vi "Excel - Read Array.vi"(6 "Cluster":T1={"start (-1, -1)"={"row"=-1, "column"=-1}, "end (-1, -1)"={"row"=-1, "column"=-1}}, 7 "name (\"\")":string, 8 "Path":path, 9 "worksheet index (0)":i32) -> (0 "False":bool, 2 "Element 1":string[][](array[string]))   [LabVIEW 2015]
uses:
  <vilib>/addons/_office/excel.llb/Excel Get Data ([str]).vi
  <vilib>/Utility/NIReport.llb/NI_report.lvclass
  <vilib>/Utility/NIReport.llb/Excel/NI_Excel.lvclass
  <vilib>/addons/_office/NI_ReportGenerationToolkit.lvlib
panel:
  in  "error in (no error)":errorcluster
  # "Select a Exel file to be Read and then Press Open"
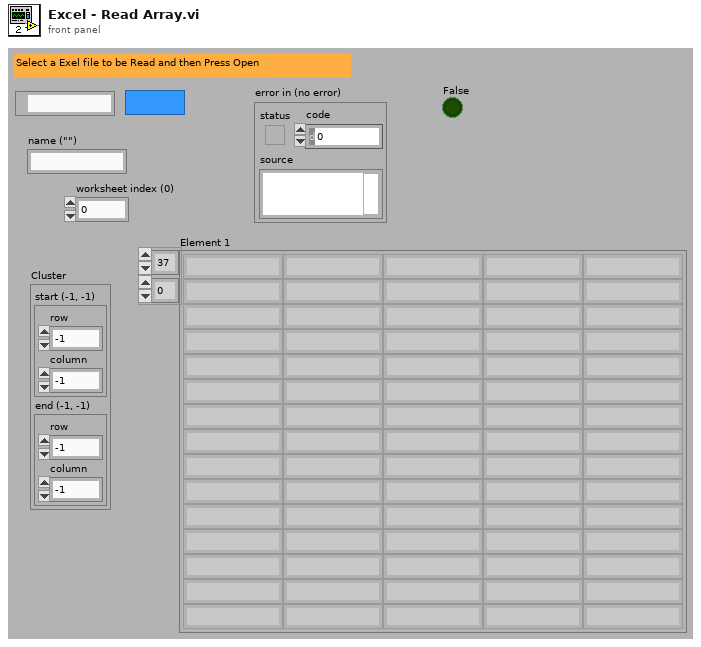
[diagram p1: front panel]
types:
  T1 = cluster{"start (-1, -1)":cluster{"row":i32, "column":i32}, "end (-1, -1)":cluster{"row":i32, "column":i32}}
  T2 = enum16{"Standard Report", "HTML", "Word", "Excel"}
  T3 = enum16{"maximized", "minimized", "normal", "no change"}
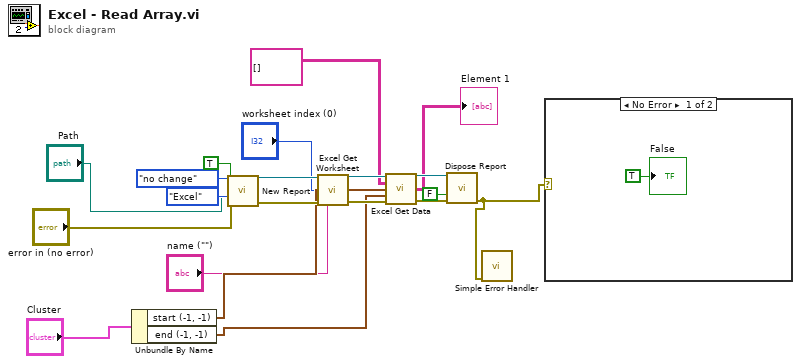
[diagram p0: block diagram]
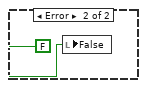
[diagram p2: hidden frame]
diagram:
  n1 = Unbundle By Name("Cluster") -> ("start (-1, -1)"=w6:cluster{"row":i32, "column":i32}, "end (-1, -1)"=w5:cluster{"row":i32, "column":i32})
  n2 = call <vilib>:"New Report.vi"("window state (normal)"=T3."no change", "display alerts? (F)"=TRUE, "report type"=T2."Excel", "template (empty)"="Path", "error in (no error)"="error in (no error)") -> ("report out"=w16:refnum<class "NI_report.lvclass">, "error out"=w15:errorcluster)  [unwired: 9 in]
  n3 = call <vilib>:"Excel Get Worksheet.vi"("report in"=w16, "worksheet index (0)"="worksheet index (0)", "error in (no error)"=w15, "name (\"\")"="name (\"\")") -> ("report out"=w14:refnum<class "NI_report.lvclass">, "error out"=w13:errorcluster)  [unwired: 10 in]
  n4 = call-poly <vilib>:"Excel Get Data.vi"("report in"=w14, "data type"=string[][] [], "start (-1, -1)"=w6, "end (-1, -1)"=w5, "error in (no error)"=w13) -> ("report out"=w10:refnum<class "NI_report.lvclass">, "data"=→"Element 1":string[][], "error out"=w11:errorcluster)  [unwired: 8 in]
  n5 = call-dynamic "Dispose Report.vi"("report in"=w10, "save changes? (F)"=FALSE, "error in (no error)"=w11) -> ("error out"=w3:errorcluster)  [unwired: 12 in]
  n6 = call <vilib>:"Simple Error Handler.vi"("error in (no error)"=w3) -> ()  [unwired: 4 in, 5 out]
  n7 = case shown="No Error" w3 {
    frame No Error {
      "False" <- TRUE ("False")
    }
    frame Error {
      n8 = local write "False"(FALSE ("False")) -> ()
    }
  }
